vi "Teardown.vi"(11 "Dev Actor in":refnum<class "Dev Actor.lvclass">=refnum) -> (3 "Dev Actor out":refnum<class "Dev Actor.lvclass">)   [LabVIEW 2021, in "Dev Actor.lvlib" / "Dev Actor.lvclass"]
uses:
  Dev Actor.lvclass
  Dev Panel/Dev Panel.lvclass
  <vilib>/jettl/jettl/Actor/Actor/Actor.lvclass
  C:/git/jettl/temp/Dev Panel/Dev Panel.lvclass
  C:/git/jettl/temp/Helper Loop/Helper Loop/Helper Loop.lvclass
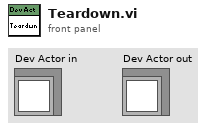
[diagram p1: front panel]
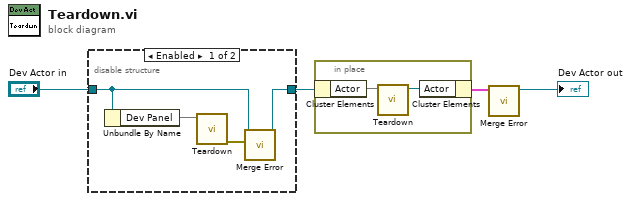
[diagram p0: block diagram]
diagram:
  n1 = disable-structure shown="Enabled" {
    disable-tunnel: "Dev Actor in" -> [w6 w9]
    disable-tunnel: [w5 w9] -> w1
    frame Enabled {
      n2 = Unbundle By Name(w6) -> ("Dev Panel"=w8)
      n3 = call "Teardown.vi"("Dev Actor Panel in"=w8) -> ("error out"=w7:errorcluster)  [unwired: 10 in]
      n4 = call-dynamic "Merge Error.vi"("Error"=w7, "Dev Actor in"=w6) -> ("Dev Actor out"=w5:refnum<class "Dev Actor.lvclass">)  [unwired: 9 in]
    }
    frame Disabled {
    }
  }
  n5 = in-place {
    n6 = in-place-cluster #1(w1) -> ("Actor"=w11)
    n7 = call-dynamic "Teardown.vi"("Teardown in"=w11) -> ("Teardown out"=w10:refnum<class "Actor.lvclass">)  [unwired: 10 in]
    n8 = in-place-cluster #1("Actor"=w10) -> (w3:cluster{})
  }
  n9 = call-dynamic "Merge Error.vi"("Dev Actor in"=w3) -> ("Dev Actor out"=→"Dev Actor out":refnum<class "Dev Actor.lvclass">)  [unwired: 10 in]
